vi "h5_write_cluster_params.vi"(7 "object name":string, 8 "error in (no error)":errorcluster, 10 "cluster":variant, 11 "h5 ref":T1 format="%.0x") -> (0 "error out":errorcluster, 3 "dup h5 ref":T1 format="%.0x")   [LabVIEW 2015]
uses:
  <vilib>/addons/h5labview2/base/hid_t.ctl
  <vilib>/Utility/Data Type/Type Definitions/Data Type.ctl
  <vilib>/addons/h5labview2/attrib/H5A.lvlib
  <vilib>/Utility/Data Type/NI_Data Type.lvlib
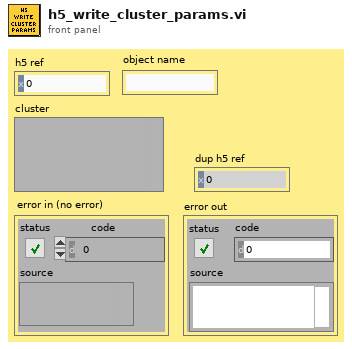
[diagram p1: front panel]
types:
  T1 = typedef "hid_t.ctl" = i32
  T2 = typedef "NI_Data Type.lvlib/Data Type.ctl" = enum8{"Invalid Type", "Void", "I8", "I16", "I32", "I64", "U8", "U16", "U32", "U64", "Single Float", "Double Float", "Extended Float", "Single Complex", "Double Complex", "Extended Complex", "Enum U8", "Enum U16", "Enum U32", "Enum U64", "Single Float With Unit", "Double Float With Unit", "Extended Float With Unit", "Single Complex with Unit", "Double Complex with Unit", "Extended Complex with Unit", "Boolean", "String", "Path", "Picture", "Tag", "Array", "Cluster", "Variant", "LV Variant", "Waveform", "Timestamp", "Digital Waveform", "Digital Data", "ExpressData", "Refnum", "External Data", "VI", "Poly VI", "LabVIEW Class Instance", "Fixed Point"}
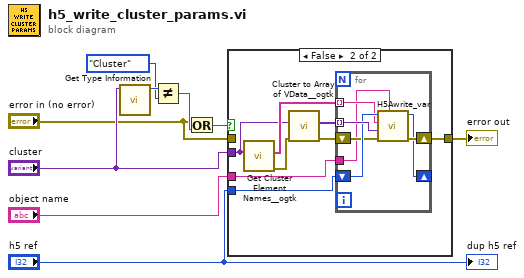
[diagram p0: block diagram]
diagram:
  n1 = call <vilib>:"Get Type Information.vi"("Variant"="cluster") -> ("Type"=w7:T2)  [unwired: 6 in, 4 out]
  n2 = Not Equal?(x=w7, y=Data_Type."Cluster" ("Type")) -> (x != y?=w5:bool)
  n3 = Or(x="error in (no error)", y=w5) -> (x .or. y?=w4:bool)
  n4 = case shown="False" w4 {
    tunnel: "cluster" -> [_ w15]
    tunnel: "h5 ref" -> [_ w14]
    tunnel: [w10 w12] -> w3
    tunnel: "error in (no error)" -> [w10 _]
    tunnel: "object name" -> [_ w11]
    frame True {
    }
    frame False {
      n5 = call <userlib>:"Get Cluster Element Names__ogtk.vi"("Cluster"=w15) -> ("error out"=w18:errorcluster, "Element Names"=w16:string[])  [unwired: 9 in]
      n6 = call <userlib>:"Cluster to Array of VData__ogtk.vi"("error in (no error)"=w18, "Cluster"=w15) -> ("error out"=w13:errorcluster, "Array of VData"=w17:variant[])  [unwired: 8 in]
      n7 = for {
        tunnel: w17 -> [w25] mode=indexing
        tunnel: w16 -> [w23] mode=indexing
        shift-right: [w21] -> w12
        shift-left: w13 -> [w22]
        shift-right: [w20] -> _
        shift-left: w14 -> [w24]
        tunnel: w11 -> [w19]
        n8 = call <vilib>:"H5Awrite_var.vi"("object name"=w19, "error in (no error)"=w22, "data"=w25, "attrib name"=w23, "ref in"=w24) -> ("error out"=w21:errorcluster, "ref out"=w20:T1)  [unwired: 4 in, 1 out]
      }
    }
  }
  "error out" <- w3
  "dup h5 ref" <- "h5 ref"
